vi "Plot Helper (Complex).vi"(8 "error in (no error)":errorcluster, 10 "z vector":cdb[](array[numeric]), 11 "2D Plot Class Obj Array in":refnum<class "2D Plot Datatype.lvclass">[](array[class])) -> (0 "error out":errorcluster, 3 "2D Plot Class Obj Array out":refnum<class "2D Plot Datatype.lvclass">[](array[class]))   [LabVIEW 2017, in "2D Compass Datatype.lvclass"]
doc: "Graphs vectors that emanate from the center origin in a compass plot. Multiple references to this VI generate multiple plots on the same graph."
uses:
  <vilib>/Math Plots/2D Math Plots/2D Compass/2D Compass Datatype/2D Compass Datatype.lvclass
  <vilib>/Math Plots/2D Math Plots/2D Plot/2D Plot Datatype/2D Plot Datatype.lvclass
  e:/builds/penguin/labview/branches/2017/dev/dist/vi.lib/Math Plots/2D Math Plots/2D Plot/2D Plot Datatype/2D Plot Datatype.lvclass
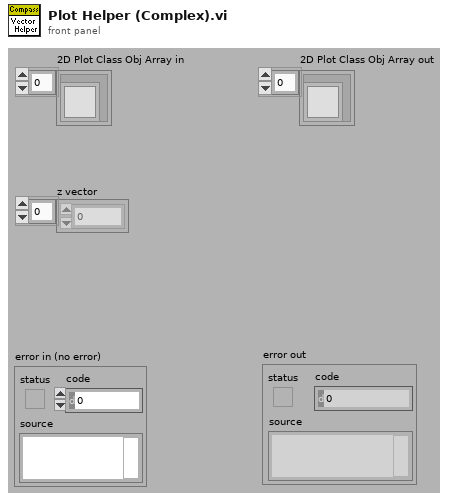
[diagram p1: front panel]
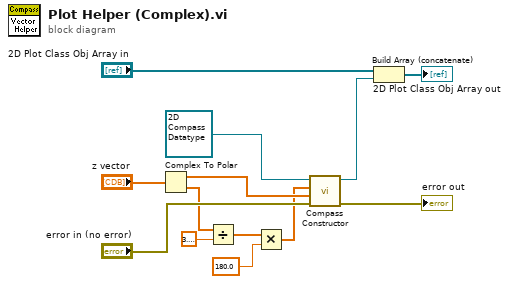
[diagram p0: block diagram]
diagram:
  n1 = Complex To Polar(r * e^(i*theta)="z vector") -> (r=w6:dbl[], theta=w4:dbl[])
  n2 = Divide(x=w4, y=3.141592653589793) -> (x/y=w3:dbl[])
  n3 = Multiply(x=w3, y=180.0) -> (x*y=w2:dbl[])
  n4 = call <vilib>:"Compass Constructor.vi"("error in (no error)"="error in (no error)", "radius vector"=w6, "theta vector"=w2, "2D Compass Datatype.lvclass in"=refnum<class "2D Compass Datatype.lvclass"> refnum ("3D Quiver Datatype.lvclass in")) -> ("error out"=→"error out":errorcluster, "2D Compass Datatype.lvclass out"=w9:refnum<class "2D Compass Datatype.lvclass">)  [unwired: 1 in, 5 out]
  n5 = Build Array (concatenate)("2D Plot Class Obj Array in", w9) -> (→"2D Plot Class Obj Array out":refnum<class "2D Plot Datatype.lvclass">[])
